vi "OFDM RX.vi"(0 "Waveform":waveform(dbl), 1 "Samples/Symbol":i32) -> (2 "Complex Waveform":T1={"t0"=0.0, "dt"=1.0, "Y"=[]} {"Y" format="%.3f"; "dt" format="%^.2e"; "t0" format="%.4f"}, 3 "Out - Waveform":waveform(dbl), 4 "Subcarriers Received":i32, 5 "Out  - Digital Subcarriers":cdb[](array[numeric]))   [LabVIEW 2018]
uses:
  <vilib>/addons/Modulation/Analog/controls/Complex Data Waveform.ctl
  <vilib>/Analysis/2dsp.llb/Real FFT.vi
  <vilib>/Analysis/NI_AALPro.lvlib
  <vilib>/addons/Modulation/niAMT.lvlib
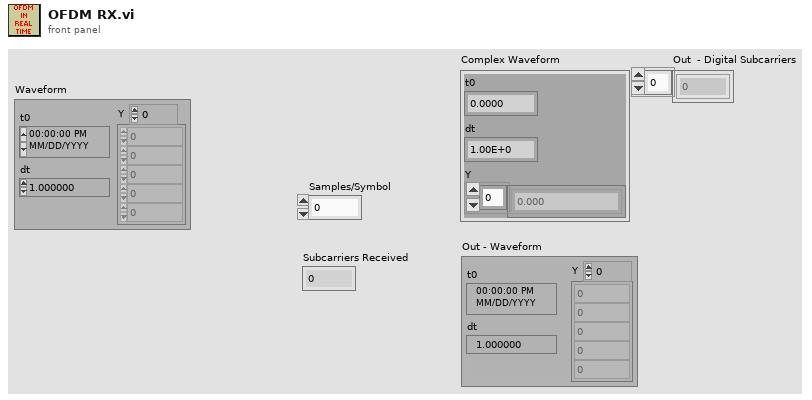
[diagram p1: front panel]
types:
  T1 = typedef "niAMT.lvlib/Complex Data Waveform.ctl" = cluster{"t0":dbl, "dt":dbl, "Y":cdb[]}
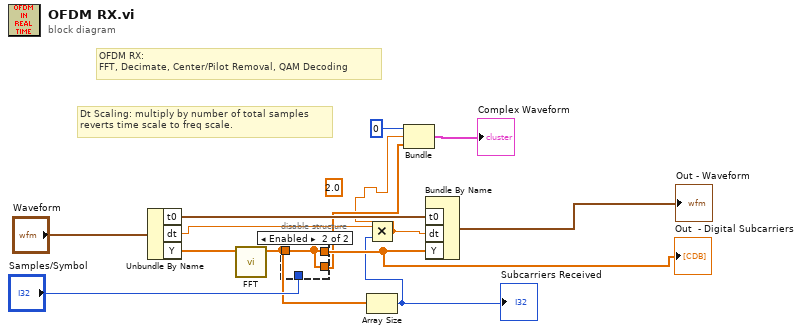
[diagram p0: block diagram]
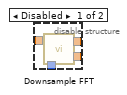
[diagram p2: hidden frame]
diagram:
  (unwired) 2.0 ("x")
  # "Dt Scaling: multiply by number of total samples\nreverts time scale to freq scale."
  # "OFDM RX:\nFFT, Decimate, Center/Pilot Removal, QAM Decoding"
  n1 = Unbundle By Name("Waveform") -> ("t0"=w8:timestamp, "dt"=w4:dbl, "Y"=w12:dbl[])
  n2 = call-poly <vilib>:"FFT.vi"("X"=w12) -> ("FFT {X}"=w2:cdb[])  [unwired: 9 in, 1 out]
  n3 = disable-structure shown="Enabled" {
    disable-tunnel: "Samples/Symbol" -> [w17 _]
    disable-tunnel: [w16 w18] -> w6
    disable-tunnel: [w15 w18] -> w5
    disable-tunnel: w2 -> [w14 w18]
    frame Disabled {
      n4 = call "Downsample FFT.vi"("Samples/Symbol"=w17, "FFT Received"=w14) -> ("FFT Downsampled (2SPS)"=w15:cdb[], "FFT Downsampled"=w16:cdb[])
    }
    frame Enabled {
    }
  }
  "Out  - Digital Subcarriers" <- w6
  n5 = Array Size(array=w2) -> (size(s)=w3:i32)
  "Subcarriers Received" <- w3
  n6 = Multiply(x=w4, y=w3) -> (x*y=w1:dbl)
  n7 = Bundle(0, w1, "FFT {X}"=w5) -> (→"Complex Waveform":cluster{i32, dbl, "FFT {X}":cdb[]})  [unwired: 1 in]
  n8 = Bundle By Name("t0"=w8, "dt"=w1, "Y"=w6) -> (→"Out - Waveform":waveform(cdb))  [unwired: 1 in]
